vi "Read out IMON.vi"(4 "get more?":bool, 5 "All Channels (T)":bool=TRUE, 7 "Channel":u8, 8 "error in (no error)":errorcluster, 11 "BoardHandle":T2) -> (0 "error out":errorcluster, 1 "IMon constants":T1(array[cluster]), 2 "IMon values (uA)":dbl[](array[numeric]) format="%.2f", 3 "BoardHandle out":T2)   [LabVIEW 2019, in "CAEN PSM.lvlib"]
doc: "This function returns Imon value"
uses:
  CAEN PSM.lvlib
  Private/BoardHandle.ctl
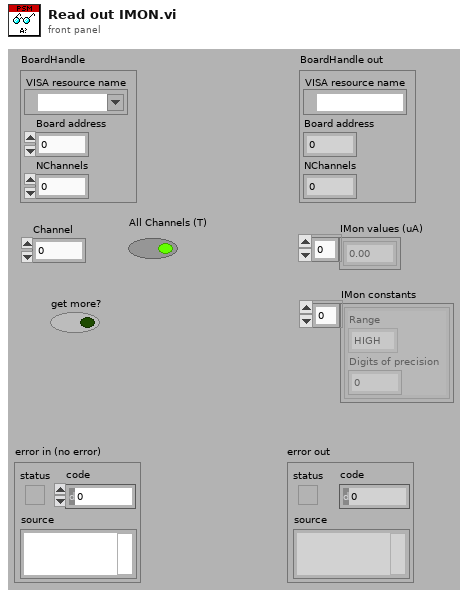
[diagram p1: front panel]
types:
  T1 = cluster{"Range":enum16{"HIGH", "LOW"}, "Digits of precision":i32}[]
  T2 = typedef "CAEN PSM.lvlib/BoardHandle.ctl" = cluster{"VISA resource name":refnum<visa-resource-name>, "Board address":u8, "NChannels":u8}
  T3 = cluster{"Range":enum16{"HIGH", "LOW"}, "Digits of precision":i32}
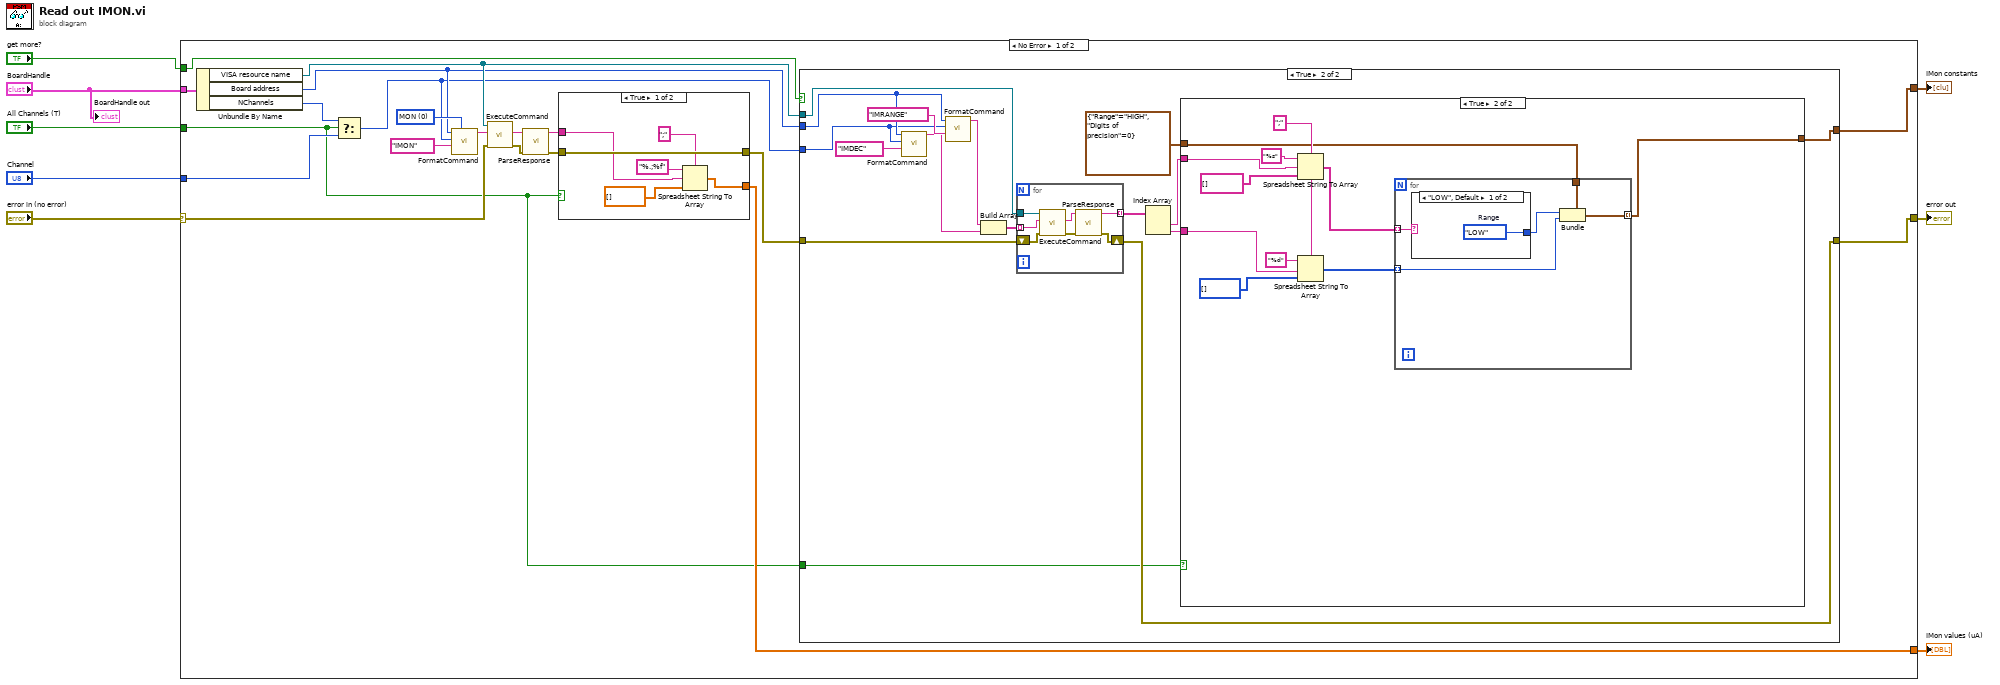
[diagram p0: block diagram]
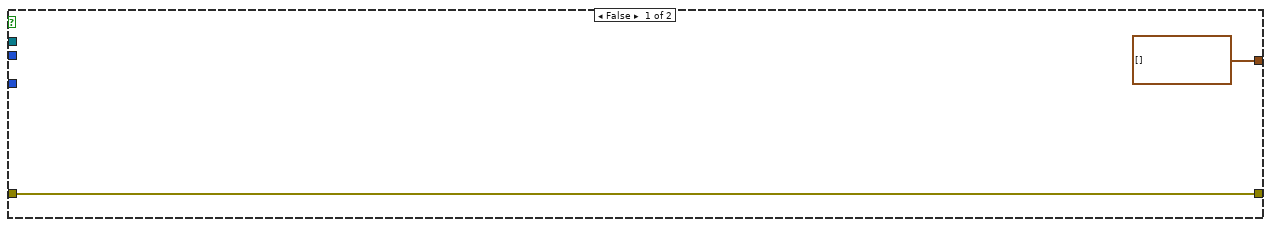
[diagram p2: hidden frame]
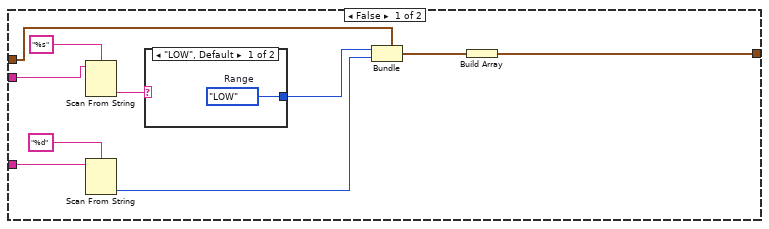
[diagram p3: hidden frame]
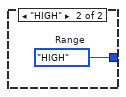
[diagram p4: hidden frame]
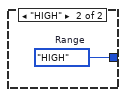
[diagram p5: hidden frame]
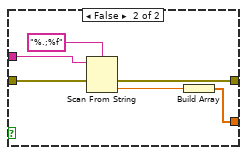
[diagram p6: hidden frame]
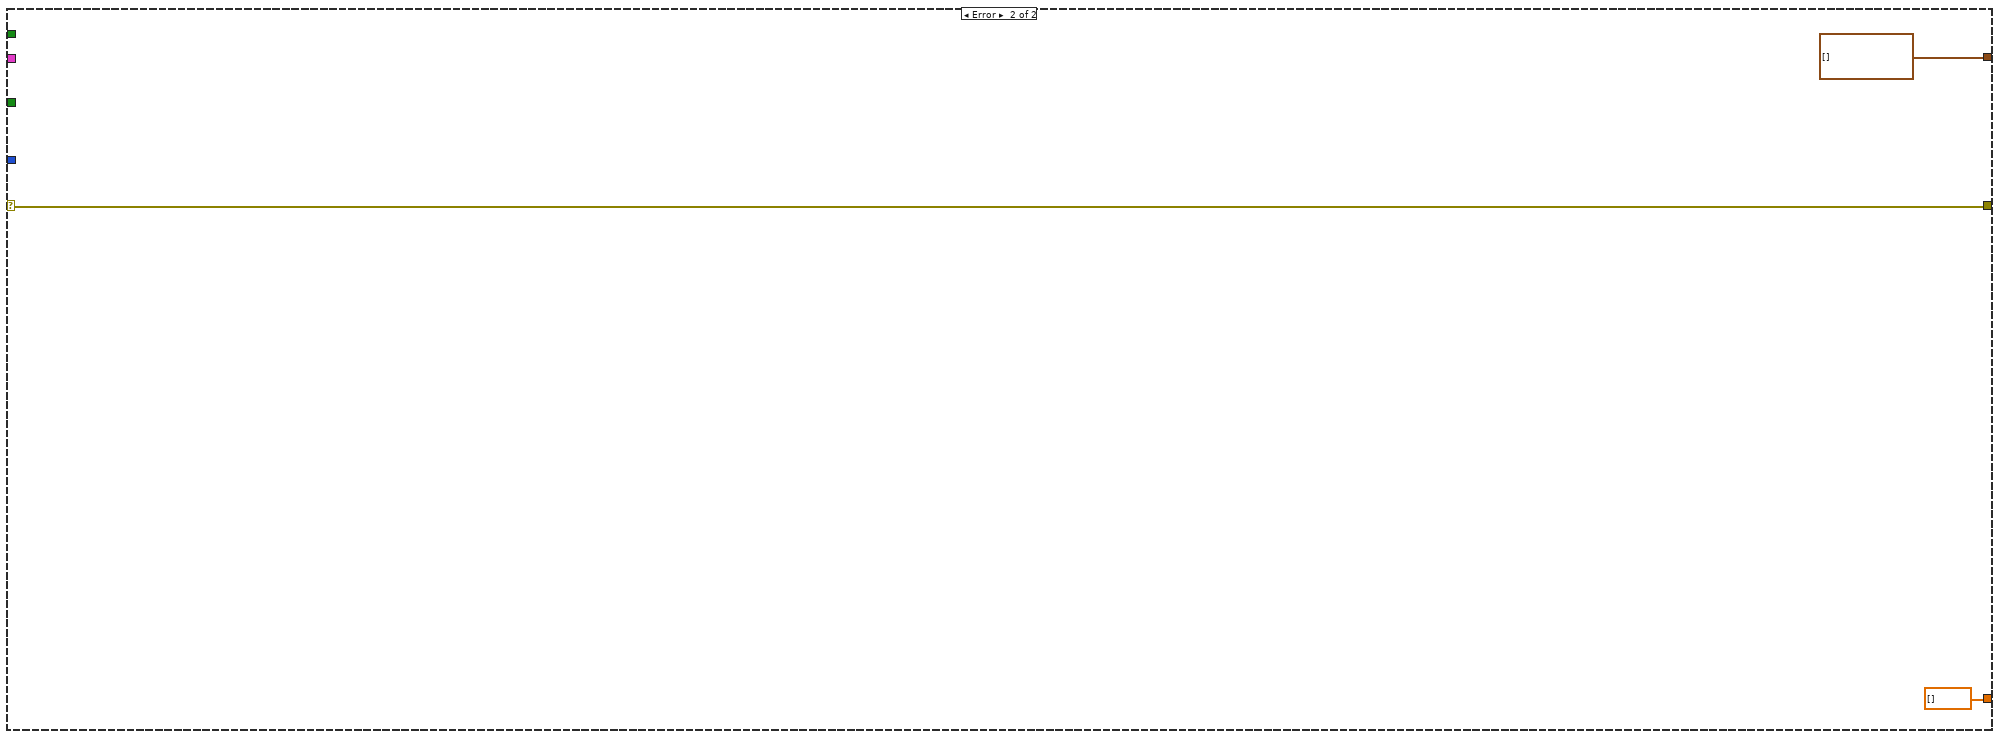
[diagram p7: hidden frame]
diagram:
  n1 = case shown="No Error" "error in (no error)" {
    selector: "error in (no error)" -> [w22 w98]
    tunnel: "All Channels (T)" -> [w9 _]
    tunnel: "Channel" -> [w27 _]
    tunnel: [w11 w98] -> w5
    tunnel: "BoardHandle" -> [w23 _]
    tunnel: [w17 dbl[] [] ("Trip value(s) s")] -> w3
    tunnel: "get more?" -> [w16 _]
    tunnel: [w10 T1 []] -> w1
    frame No Error {
      w28 = u8 0 items=["MON", "SET"] ("CMD")
      n2 = Unbundle By Name(w23) -> ("VISA resource name"=w15:refnum<visa-resource-name>, "Board address"=w14:u8, "NChannels"=w20:u8)
      n3 = Select(t=w20, s=w9, f=w27) -> (s? t:f=w13:u8)
      n4 = call "FormatCommand.vi"("CMD (MON)"=w28, "PAR"="IMON", "CH"=w13, "BD (0)"=w14) -> ("cmd"=w26:string)  [unwired: 7 in]
      n5 = call "ExecuteCommand.vi"("error in (no error)"=w22, "Command"=w26, "VISA resource name"=w15) -> ("error out"=w25:errorcluster, "Response"=w24:string)  [unwired: 6 in, 1 out]
      n6 = call "ParseResponse.vi"("error in (no error)"=w25, "Response"=w24) -> ("error out"=w18:errorcluster, "val"=w19:string)  [unwired: 6 in, 2 out]
      n7 = case shown="True" w9 {
        tunnel: w19 -> [w84 w95]
        tunnel: w18 -> [w89 w93]
        tunnel: [w89 w92] -> w12
        tunnel: [w85 w90] -> w17
        frame True {
          n8 = Spreadsheet String To Array(delimiter (Tab)=";", format string="%.;%f", spreadsheet string=w84, array type (2D Dbl)=dbl[] []) -> (array=w85:dbl[])
        }
        frame False {
          n9 = Scan From String(format string="%.;%f", input string=w95, error in=w93) -> (error out=w92:errorcluster, output 1=w91:dbl)  [unwired: 2 in, 2 out]
          n10 = Build Array(w91) -> (w90:dbl[])
        }
      }
      n11 = case shown="True" w16 {
        tunnel: w12 -> [w30 w38]
        tunnel: [w30 w37] -> w11
        tunnel: w15 -> [_ w41]
        tunnel: w14 -> [_ w40]
        tunnel: w13 -> [_ w39]
        tunnel: [T1 [] w32] -> w10
        tunnel: w9 -> [_ w31]
        frame False {
        }
        frame True {
          n12 = call "FormatCommand.vi"("PAR"="IMDEC", "CH"=w39, "BD (0)"=w40) -> ("cmd"=w42:string)  [unwired: 8 in]
          n13 = call "FormatCommand.vi"("PAR"="IMRANGE", "CH"=w39, "BD (0)"=w40) -> ("cmd"=w43:string)  [unwired: 8 in]
          n14 = Build Array(w43, w42) -> (w44:string[])
          n15 = for {
            tunnel: w44 -> [w83] mode=indexing
            tunnel: w41 -> [w82]
            shift-right: [w80] -> w37
            shift-left: w38 -> [w81]
            tunnel: [w77] -> w36 mode=indexing
            n16 = call "ExecuteCommand.vi"("error in (no error)"=w81, "Command"=w83, "VISA resource name"=w82) -> ("error out"=w79:errorcluster, "Response"=w78:string)  [unwired: 6 in, 1 out]
            n17 = call "ParseResponse.vi"("error in (no error)"=w79, "Response"=w78) -> ("error out"=w80:errorcluster, "val"=w77:string)  [unwired: 6 in, 2 out]
          }
          n18 = Index Array(array=w36) -> (element #1=w35:string, element #2=w33:string)  [unwired: 2 in]
          n19 = case shown="True" w31 {
            tunnel: w35 -> [w56 w64]
            tunnel: w33 -> [w53 w61]
            tunnel: T3 {"Range"=enum."HIGH", "Digits of precision"=0} -> [w52 w66]
            tunnel: [w49 w65] -> w32
            frame False {
              n20 = Scan From String(format string="%s", input string=w56) -> (output 1=w48:string)  [unwired: 3 in, 3 out]
              n21 = Scan From String(format string="%d", input string=w53) -> (output 1=w51:i32)  [unwired: 3 in, 3 out]
              n22 = case shown="\"LOW\", Default" w48 {
                tunnel: [w57 w58] -> w47
                frame "LOW", Default {
                  w57 = enum16{"HIGH", "LOW"}."LOW"  # Range
                }
                frame "HIGH" {
                  w58 = enum16{"HIGH", "LOW"}."HIGH"  # Range
                }
              }
              n23 = Bundle(cluster=w52, "Range"=w47, "Digits of precision"=w51) -> (w50:T3)
              n24 = Build Array(w50) -> (w49:T1)
            }
            frame True {
              w67 = ";" ("delimiter (Tab)")
              n25 = Spreadsheet String To Array(delimiter (Tab)=w67, format string="%s", spreadsheet string=w64, array type (2D Dbl)=string[] []) -> (array=w62:string[])
              n26 = Spreadsheet String To Array(delimiter (Tab)=w67, format string="%d", spreadsheet string=w61, array type (2D Dbl)=i32[] []) -> (array=w59:i32[])
              n27 = for {
                tunnel: w66 -> [w74]
                tunnel: [w73] -> w65 mode=indexing
                tunnel: w62 -> [w72] mode=indexing
                tunnel: w59 -> [w70] mode=indexing
                n28 = case shown="\"LOW\", Default" w72 {
                  tunnel: [w75 w76] -> w71
                  frame "LOW", Default {
                    w75 = enum16{"HIGH", "LOW"}."LOW"  # Range
                  }
                  frame "HIGH" {
                    w76 = enum16{"HIGH", "LOW"}."HIGH"  # Range
                  }
                }
                n29 = Bundle(cluster=w74, "Range"=w71, "Digits of precision"=w70) -> (w73:T3)
              }
            }
          }
        }
      }
    }
    frame Error {
    }
  }
  "error out" <- w5
  "IMon values (uA)" <- w3
  "IMon constants" <- w1
  "BoardHandle out" <- "BoardHandle"
